vi "Draw Pattern Layer.vi"() -> ()   [LabVIEW 2021]
doc: "This example allows to draw patterns in the scan control module by means of drawing lines using the mouse over the Picture control.\n\nThe Picture control covers the entire scan frame. An image of the current scan databuffer can be grabbed and pasted into the Picture control.\n\nWhat it is drawn in the Picture control (clicking and dragging the mouse to the point where the line finishes) is mirrored in the scan control module.\n\n- Nanonis Programming Interface -"
uses:
  Nanonis Prog Interface.lvlib
panel:
  in  "Fwd/Bwd (T=Fwd)":bool=TRUE
  in  "Clear Lines":bool
  out "Databuffer image":picture
  in  "Channel":u8(ring) items=["Current (A)"=0, "Input 5 (V)"=4, "Z (m)"=14, "Phase (deg)"=16, "Amplitude (m)"=17, "Frequency Shift (Hz)"=18, "Excitation (V)"=19]
  in  "Grab image":bool
  in  "Undo":bool
  in  "Pen Color (in Scan Module)":u32(colorbox)=61225
  in  "Clear All":bool
  out "Initial mouse position":cluster{"X":i32, "Y":i32}
  in  "Pen Color (in Picture)":u32(colorbox)=3381759
  out "Draw??":bool
  in  "stop":bool
  in  "Pen Attributes":T1={"Width"=2, "Style"=enum."Solid"}
  out "Picture":picture
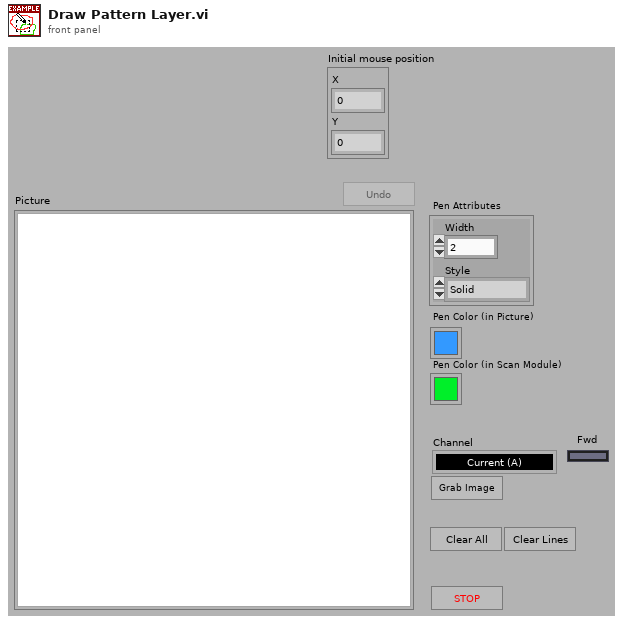
[diagram p1: front panel]
types:
  T1 = cluster{"Width":u16, "Style":enum32{"Solid", "Dash", "Dot", "DashDot", "DashDotDot"}}
  T2 = typedef "LVMouseTypeDef.ctl" = cluster{"Mouse Position":cluster{"X":i32, "Y":i32}, "Mouse Modifiers":cluster{"Button Down":bool, "Shift Mod":bool, "Menu Mod":bool, "Option Mod":bool}}
  T3 = cluster{"Start":cluster{"X1 (m)":sgl, "Y1 (m)":sgl}, "End":cluster{"X2 (m)":sgl, "Y2 (m)":sgl}, "Line Color":u32, "Visible":bool}[]
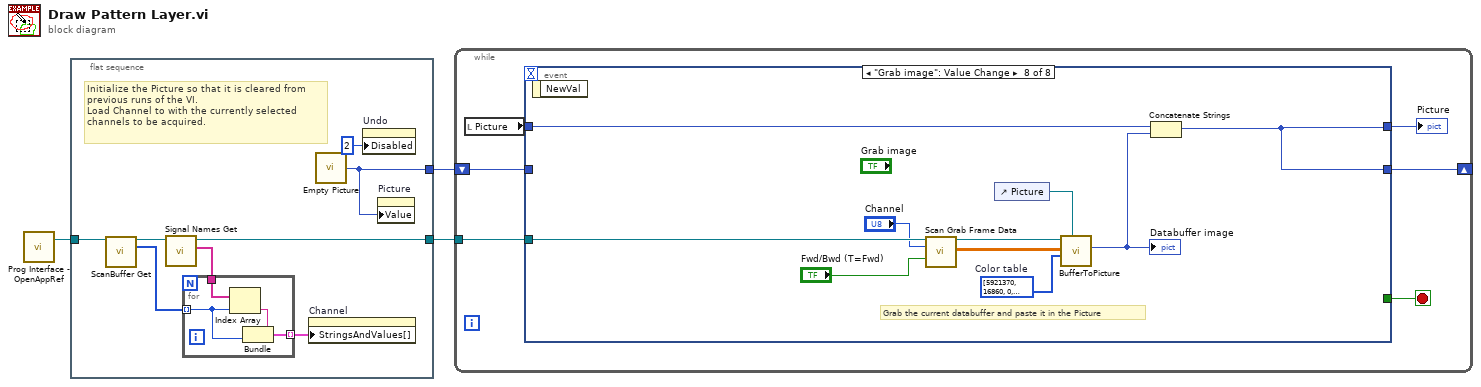
[diagram p0: block diagram]
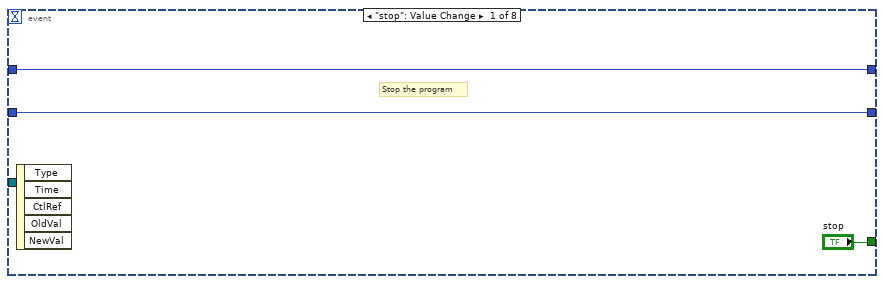
[diagram p2: hidden frame]
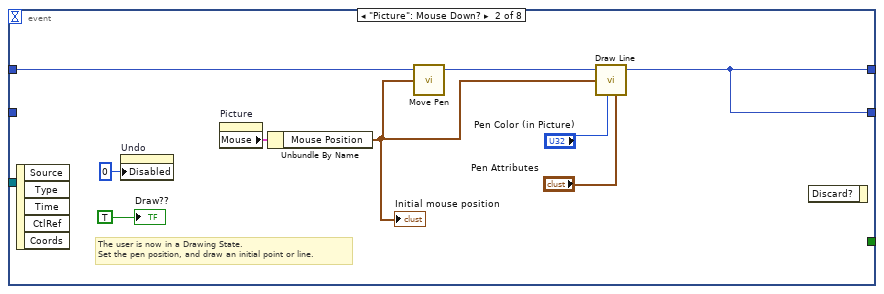
[diagram p3: hidden frame]
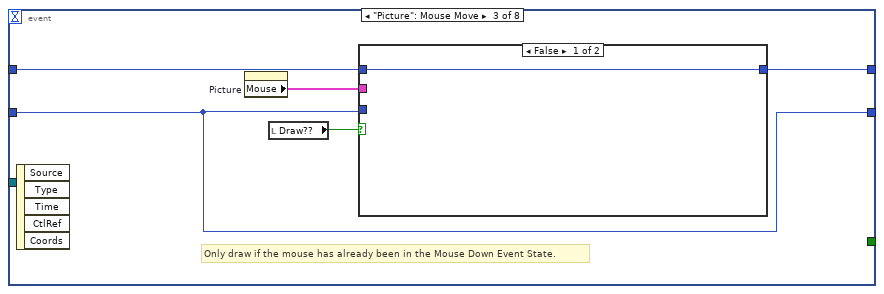
[diagram p4: hidden frame]
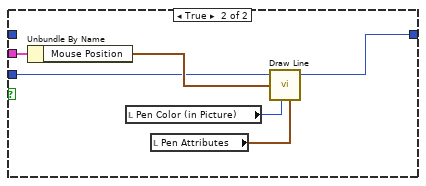
[diagram p5: hidden frame]
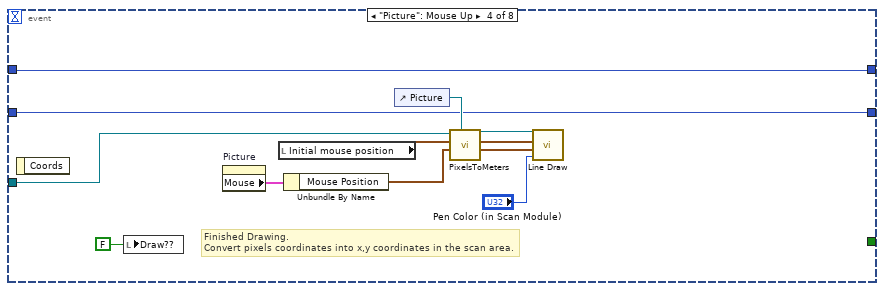
[diagram p6: hidden frame]
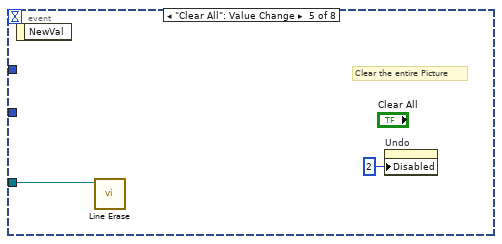
[diagram p7: hidden frame]
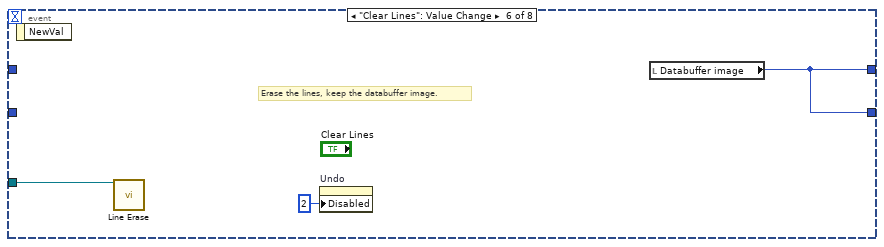
[diagram p8: hidden frame]
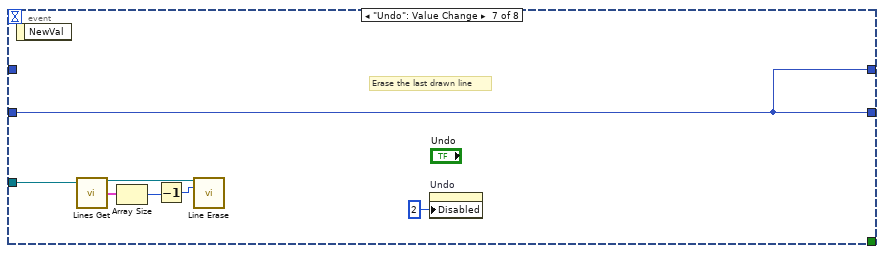
[diagram p9: hidden frame]
diagram:
  n1 = call <userlib>:"Prog Interface - OpenAppRef.vi"() -> ("Application reference"=w2:refnum<vi>)  [unwired: 6 in, 1 out]
  n2 = flat-sequence {
    tunnel: [w11] -> w3
    tunnel: w2 -> [w8]
    tunnel: [w6] -> w1
    frame #0 {
      # "Initialize the Picture so that it is cleared from previous runs of the VI.\nLoad Channel to with the currently selected channels to be acquired."
      n3 = call <userlib>:"ScanBuffer Get.vi"("Application ref in"=w8) -> ("Application ref out"=w5:refnum<vi>, "Channels indexes (0-127)"=w9:i32[])  [unwired: 10 in, 3 out]
      n4 = call <userlib>:"Signal Names Get.vi"("Application ref in"=w5) -> ("Signals Names"=w4:string[], "Application ref out"=w6:refnum<vi>)  [unwired: 6 in, 1 out]
      n5 = for {
        tunnel: w9 -> [w13] mode=indexing
        tunnel: w4 -> [w15]
        tunnel: [w12] -> w7 mode=indexing
        n6 = Index Array(array=w15, index=w13) -> (element=w14:string)
        n7 = Bundle("String"=w14, "Numeric"=w13) -> (w12:cluster{"String":string, "Numeric":i32})  [unwired: 1 in]
      }
      n8 = property on="Channel" class="Ring (strict)"("StringsAndValues[]"=w7) -> ()  [unwired: 2 in, 2 out]
      n9 = call "Empty Picture"() -> ("empty picture"=w11:picture)
      n10 = property on="Undo" class="Bool"("Disabled"=u8 2) -> ()  [unwired: 2 in, 2 out]
      n11 = property on="Picture" class="Pict"("Value"=w11) -> ()  [unwired: 2 in, 2 out]
    }
  }
  n12 = while {
    shift-right: [w19] -> _
    shift-left: w3 -> [w18]
    tunnel: w1 -> [w16]
    stop <- w21 stop-if-true
    n13 = local read "Picture"() -> (w20:picture)
    n14 = event shown="[7] \"Grab image\": Value Change" {
      selector: _ -> [_ _ _ _ _ _ _ _]
      dyn-events: _ -> [_ _ _ _ _ _ _ _]
      timeout: _ -> [_ _ _ _ _ _ _ _]
      tunnel: ["stop" _ _ _ _ _ _ _] -> w21
      tunnel: [w23 w29 w36 w46 _ w62 w64 w76] -> w17
      tunnel: w20 -> [w23 w31 w35 w46 _ _ _ w77]
      tunnel: [w22 w29 w34 w47 _ w62 w64 w76] -> w19
      tunnel: w18 -> [w22 _ w34 w47 _ _ w64 _]
      tunnel: w16 -> [_ _ _ w52 w59 w61 w68 w79]
      event "stop": Value Change {
        # "Stop the program"
        n15 = event-data() -> ()  [unwired: 1 in, 5 out]
      }
      event "Picture": Mouse Down? {
        # "The user is now in a Drawing State.\nSet the pen position, and draw an initial point or line."
        n16 = event-data() -> ()  [unwired: 1 in, 5 out]
        n17 = property on="Undo" class="Bool"("Disabled"=u8 0) -> ()  [unwired: 2 in, 2 out]
        n18 = property on="Picture" class="Pict"() -> ("Mouse"=w33:T2)  [unwired: 2 in, 2 out]
        n19 = Unbundle By Name(w33) -> ("Mouse Position"=w28:cluster{"X":i32, "Y":i32})
        "Initial mouse position" <- w28
        n20 = call <vilib>:"Move Pen.vi"("new position"=w28, "picture"=w31) -> ("new picture"=w30:picture)  [unwired: 3 in]
        n21 = call <vilib>:"Draw Line.vi"("picture"=w30, "end point"=w28, "color(black)"="Pen Color (in Picture)", "pen"="Pen Attributes") -> ("new picture"=w29:picture)  [unwired: 5 in]
        n22 = event-data() -> ()  [unwired: 2 in, 1 out]
        "Draw??" <- TRUE ("Draw??")
      }
      event "Picture": Mouse Move {
        # "Only draw if the mouse has already been in the Mouse Down Event State."
        n23 = event-data() -> ()  [unwired: 1 in, 5 out]
        n24 = property on="Picture" class="Pict"() -> ("Mouse"=w37:T2)  [unwired: 2 in, 2 out]
        n25 = local read "Draw??"() -> (w38:bool)
        n26 = case shown="False" w38 {
          tunnel: w35 -> [w39 _]
          tunnel: w37 -> [_ w45]
          tunnel: [w39 w43] -> w36
          tunnel: w34 -> [_ w42]
          frame False {
          }
          frame True {
            n27 = Unbundle By Name(w45) -> ("Mouse Position"=w44:cluster{"X":i32, "Y":i32})
            n28 = local read "Pen Color (in Picture)"() -> (w40:u32)
            n29 = local read "Pen Attributes"() -> (w41:T1)
            n30 = call <vilib>:"Draw Line.vi"("picture"=w42, "end point"=w44, "color(black)"=w40, "pen"=w41) -> ("new picture"=w43:picture)  [unwired: 5 in]
          }
        }
      }
      event "Picture": Mouse Up {
        # "Finished Drawing.\nConvert pixels coordinates into x,y coordinates in the scan area."
        n31 = event-data() -> ()  [unwired: 1 in, 1 out]
        n32 = local write "Draw??"(FALSE ("Draw??")) -> ()
        n33 = property on="Picture" class="Pict"() -> ("Mouse"=w56:T2)  [unwired: 2 in, 2 out]
        n34 = local read "Initial mouse position"() -> (w50:cluster{"X":i32, "Y":i32})
        n35 = Unbundle By Name(w56) -> ("Mouse Position"=w48:cluster{"X":i32, "Y":i32})
        n36 = control-ref of="Picture"() -> (w51:refnum<vi>)
        n37 = call "PixelsToMeters.vi"("Pict Refnum"=w51, "End mouse position (px)"=w48, "Initial mouse position (px)"=w50, "Application reference in"=w52) -> ("End mouse position (m)"=w49:cluster{sgl, sgl}, "Initial mouse position (m)"=w54:cluster{sgl, sgl}, "Application reference out"=w53:refnum<vi>)  [unwired: 5 in]
        n38 = call <userlib>:"Line Draw.vi"("Application ref in"=w53, "Start Point Coordinates"=w54, "End Point Coordinates"=w49, "Color"="Pen Color (in Scan Module)") -> ()  [unwired: 10 in, 2 out]
      }
      event "Clear All": Value Change {
        # "Clear the entire Picture"
        n39 = event-data() -> ()  [unwired: 1 in, 1 out]
        n40 = call <userlib>:"Line Erase.vi"("Application ref in"=w59) -> ()  [unwired: 13 in, 2 out]
        n41 = property on="Undo" class="Bool"("Disabled"=u8 2) -> ()  [unwired: 2 in, 2 out]
      }
      event "Clear Lines": Value Change {
        # "Erase the lines, keep the databuffer image."
        n42 = event-data() -> ()  [unwired: 1 in, 1 out]
        n43 = call <userlib>:"Line Erase.vi"("Application ref in"=w61) -> ()  [unwired: 13 in, 2 out]
        n44 = property on="Undo" class="Bool"("Disabled"=u8 2) -> ()  [unwired: 2 in, 2 out]
        n45 = local read "Databuffer image"() -> (w62:picture)
      }
      event "Undo": Value Change {
        # "Erase the last drawn line"
        n46 = event-data() -> ()  [unwired: 1 in, 1 out]
        n47 = call <userlib>:"Lines Get.vi"("Application ref in"=w68) -> ("Application ref out"=w69:refnum<vi>, "Lines"=w67:T3)  [unwired: 12 in, 1 out]
        n48 = Array Size(array=w67) -> (size(s)=w65:i32)
        n49 = Decrement(x=w65) -> (x-1=w66:i32)
        n50 = call <userlib>:"Line Erase.vi"("Application ref in"=w69, "Line index (-1=All lines)"=w66) -> ()  [unwired: 12 in, 2 out]
        n51 = property on="Undo" class="Bool"("Disabled"=u8 2) -> ()  [unwired: 2 in, 2 out]
      }
      event "Grab image": Value Change {
        w71 = u32[] [5921370, 16860, 0, 262400, 459008, 721408, 983808, 1180416, 1442816, 1705216, 1901824, 2164224, 2426368, 2623232, 2885632, 3147776, 3344640, 3607040, 3869184, 4131584, 4328448, 4590592, 4852992, 5049856, 5312000, 5574400, 5771264, 6033408, 6295808, 6492416, 6754816, 7017216, 7213824, 7476224, 7738624, 7935232, 8197632, 8460032, 8656640, 8919040, 9181440, 9378048, 9640448, 9902592, 10099456, 10361856, 10624000, 10820864, 11083264, 11345408, 11542272, 11804672, 12066816, 12329216, 12526080, 12788224, 13050624, 13247488, 13509632, 13772032, 13968640, 14231040, 14493440, 14690048, 14952448, 15214848, 15411456, 15673856, 15674112, 15740160, 15740416, 15740928, 15741184, 15806976, 15807488, 15807744, 15808256, 15874048, 15874560, 15874816, 15875072, 15941120, 15941376, 15941888, 15942144, 16007936, 16008448, 16008704, 16074752, 16075008, 16075264, 16075776, 16141568, 16142080, 16142336, 16142592, 16208640, 16208896, 16209408, 16209664, 16275712, 16275968, 16276224, 16276736, 16342528, 16343040, 16343296, 16343552, 16409600, 16409856, 16410368, 16476160, 16476416, 16476928, 16477184, 16543232, 16543488, 16543744, 16544256, 16610048, 16610560, 16610816, 16611328, 16677120, 16677376, 16677888, 16678144, 16744192, 16744448, 16744960, 16745472, 16745984, 16746496, 16746752, 16747264, 16747776, 16748288, 16748800, 16749312, 16749824, 16750336, 16750848, 16751360, 16751616, 16752128, 16752640, 16753152, 16753664, 16754176, 16754688, 16755200, 16755712, 16755968, 16756480, 16756992, 16757504, 16758016, 16758528, 16759040, 16759552, 16760064, 16760576, 16760832, 16761344, 16761856, 16762368, 16762880, 16763392, 16763904, 16764416, 16764928, 16765440, 16765696, 16766208, 16766720, 16767232, 16767744, 16768256, 16768768, 16769280, 16769792, 16770048, 16770560, 16771072, 16771584, 16772096, 16772608, 16773120, 16773632, 16774144, 16774656, 16774912, 16775424, 16775936, 16776448, 16776960, 16776964, 16776969, 16776973, 16776977, 16776982, 16776986, 16776990, 16776995, 16776999, 16777003, 16777008, 16777012, 16777016, 16777021, 16777025, 16777029, 16777033, 16777038, 16777042, 16777046, 16777051, 16777055, 16777059, 16777064, 16777068, 16777072, 16777077, 16777081, 16777085, 16777090, 16777094, 16777098, 16777103, 16777107, 16777111, 16777116, 16777120, 16777124, 16777129, 16777133, 16777137, 16777142, 16777146, 16777150, 16777154, 16777159, 16777163, 16777167, 16777172, 16777176, 16777180, 16777185, 16777189, 16777193, 16777198, 16777202, 16777206, 16777211, 16777215, 16711680]  # Color table
        # "Grab the current databuffer and paste it in the Picture"
        n52 = event-data() -> ()  [unwired: 1 in, 1 out]
        n53 = call <userlib>:"Scan Grab Frame Data.vi"("Application ref in"=w79, "Channel index (0-127)"="Channel", "Direction: Fwd/Bwd (T=Fwd)"="Fwd/Bwd (T=Fwd)") -> ("Application ref out"=w74:refnum<vi>, "Scan frame data"=w73:sgl[][])  [unwired: 8 in, 3 out]
        n54 = control-ref of="Picture"() -> (w75:refnum<vi>)
        n55 = call <userlib>:"BufferToPicture.vi"("Pict Refnum"=w75, "Colortable"=w71, "Scan frame data"=w73, "Application ref in"=w74) -> ("Databuffer bitmap"=w72:picture)  [unwired: 6 in, 1 out]
        "Databuffer image" <- w72
        n56 = Concatenate Strings(w77, w72) -> (w76:picture)
      }
    }
    "Picture" <- w17
  }
